vi "Cleanup.vi"(8 "error in":errorcluster, 11 "Philips UI in":refnum<class "Flex UI.lvclass">) -> (0 "error out":errorcluster)   [LabVIEW 2014, in "Flex UI.lvclass"]
doc: "Cleans up after the UI.\n\nRuns EVEN IF an error has occurred upstream."
uses:
  Flex UI.lvclass
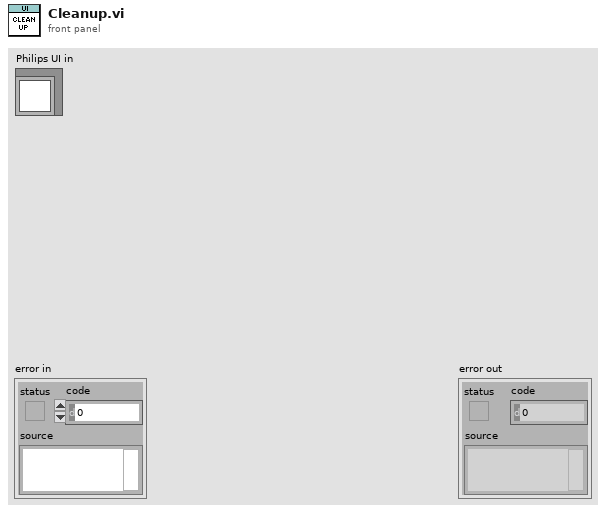
[diagram p1: front panel]
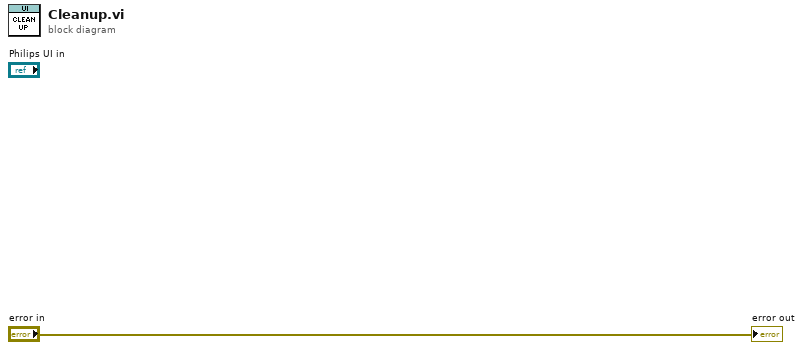
[diagram p0: block diagram]
diagram:
  "error out" <- "error in"
